vi "Read configuration.vi"(8 "error in":errorcluster, 11 "EthernetIP editor node in":refnum<class "EthernetIP editor node.lvclass">) -> (0 "error out":errorcluster, 2 "TBM configuration out":refnum<class "NISE_CEF_serializable configuration.lvclass">, 3 "EthernetIP editor node out":refnum<class "EthernetIP editor node.lvclass">)   [LabVIEW 2013, in "EthernetIP editor node.lvclass"]
uses:
  EthernetIP editor node.lvclass
  <vilib>/NI/Configuration Framework/serializable configuration/NISE_CEF_serializable configuration.lvclass
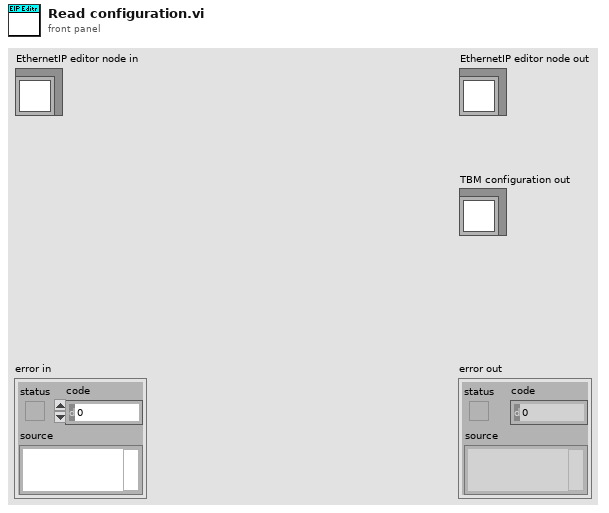
[diagram p1: front panel]
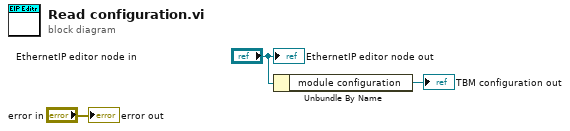
[diagram p0: block diagram]
diagram:
  n1 = Unbundle By Name("EthernetIP editor node in") -> ("module configuration"=→"TBM configuration out":refnum<class "EthernetIP configuration.lvclass">)
  "error out" <- "error in"
  "EthernetIP editor node out" <- "EthernetIP editor node in"
